vi "Read Measurement (Occupied Bandwidth).vi"(0 "VISA resource name":refnum<visa-resource-name>, 5 "Timeout (10000 ms)":i32=10000 format="%.0g", 11 "error in (no error)":errorcluster) -> (2 "Transmit Frequency Error Hz":dbl, 3 "Res BW":dbl, 4 "VISA resource name out":refnum<visa-resource-name>, 6 "Occupied Bandwidth":dbl, 8 "Spectrum Trace Points":dbl, 10 "Total Power":dbl, 13 "X DB Bandwidth":dbl, 14 "Span":dbl, 15 "error out":errorcluster)   [LabVIEW 2014, in "Agilent MXA Series.lvlib"]
doc: "Reads the measurement result from the spectrum analyzer(Occupied Bandwidth)."
uses:
  Agilent MXA Series.lvlib
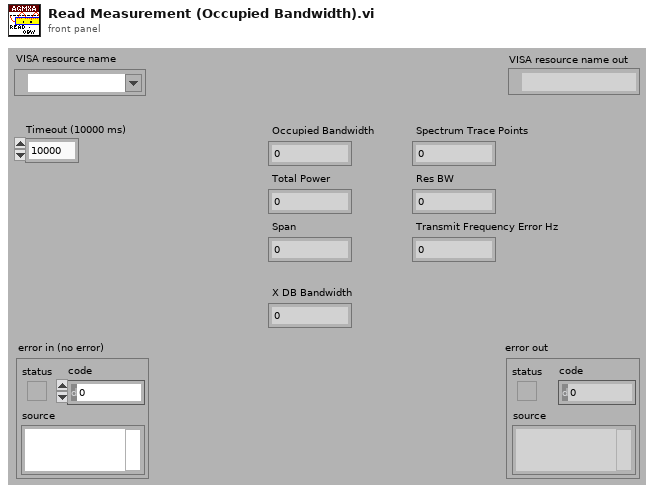
[diagram p1: front panel]
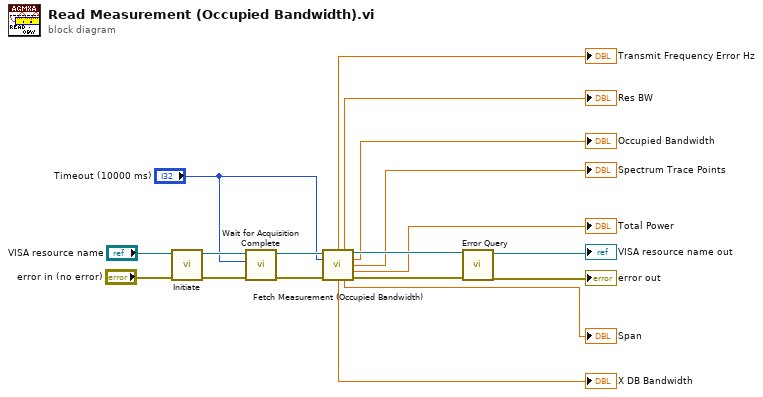
[diagram p0: block diagram]
diagram:
  n1 = call "Initiate.vi"("error in (no error)"="error in (no error)", "VISA resource name"="VISA resource name") -> ("error out"=w15:errorcluster, "VISA resource name out"=w16:refnum<visa-resource-name>)  [unwired: 8 in]
  n2 = call "Wait for Acquisition Complete.vi"("error in (no error)"=w15, "Maximum Time (10000)"="Timeout (10000 ms)", "VISA resource name"=w16) -> ("error out"=w13:errorcluster, "VISA resource name out"=w14:refnum<visa-resource-name>)  [unwired: 7 in]
  n3 = call "Fetch Measurement (Occupied Bandwidth).vi"("VISA resource name"=w14, "Timeout (10000 ms)"="Timeout (10000 ms)", "error in (no error)"=w13) -> ("Transmit Frequency Error Hz"=→"Transmit Frequency Error Hz":dbl, "Res BW"=→"Res BW":dbl, "VISA resource name out"=w12:refnum<visa-resource-name>, "Occupied Bandwidth"=→"Occupied Bandwidth":dbl, "Spectrum Trace Points"=→"Spectrum Trace Points":dbl, "Total Power"=→"Total Power":dbl, "X DB Bandwidth"=→"X DB Bandwidth":dbl, "Span"=→"Span":dbl, "error out"=w11:errorcluster)  [unwired: 4 in]
  n4 = call "Error Query.vi"("error in (no error)"=w11, "VISA resource name"=w12) -> ("error out"=→"error out":errorcluster, "VISA resource name out"=→"VISA resource name out":refnum<visa-resource-name>)  [unwired: 6 in, 2 out]
